vi "Test Never Any Inputs Fail.vi"(8 "error in (no error)":errorcluster, 11 "Test Case In":refnum<class "Expectation Message Test.lvclass">) -> (0 "error out":errorcluster, 3 "Test Case Out":refnum<class "Expectation Message Test.lvclass">)   [LabVIEW 2020, in "Expectation Message Test.lvclass"]
uses:
  Expectation Message Test.lvclass
  C:/Program Files (x86)/National Instruments/LabVIEW 2020/vi.lib/Astemes/LUnit/Test Case.lvclass
  Test Doubles/Test Interface Responsive Mock/Test Interface Mock.lvclass
  C:/git/astemes-lmock/source/Framework/Mock/Mock.lvclass
  source/Expectations/Never/Never Ignore Inputs.vi
  C:/git/astemes-lmock/tests/Test Doubles/Test Interface Responsive Mock/Test Interface Mock.lvclass
  C:/git/astemes-lmock/tests/Test Doubles/Test Interface/Test Interface.lvclass
  source/Framework/LMock API.lvlib
  source/Expectations/Never/Never.lvlib
  Expectation Test/Expectation Test.lvclass
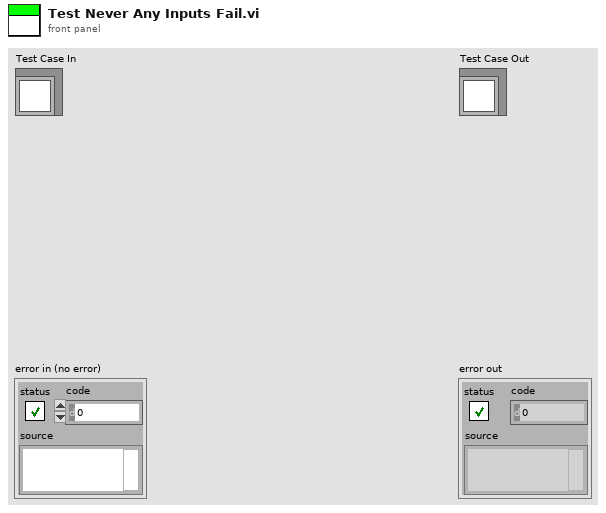
[diagram p1: front panel]
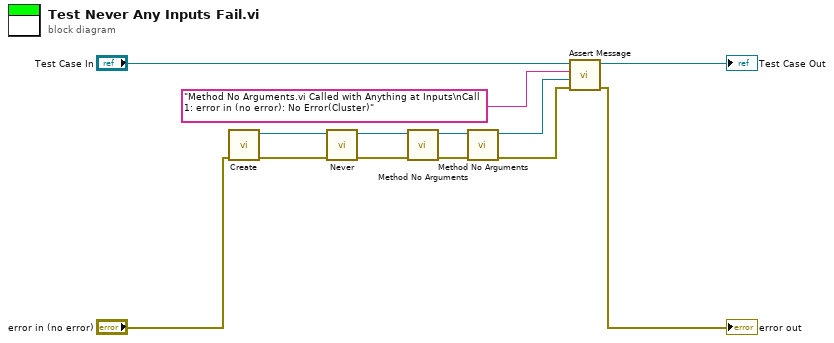
[diagram p0: block diagram]
diagram:
  n1 = call "Create.vi"("error in (no error)"="error in (no error)") -> ("error out"=w10:errorcluster, "Test Interface Mock Out"=w8:refnum<class "Test Interface Mock.lvclass">)  [unwired: 9 in]
  n2 = call-poly "Never.vi"("error in (no error)"=w10, "Mock in"=w8) -> ("error out"=w9:errorcluster, "Mock out"=w7:refnum<class "Test Interface Mock.lvclass">)  [unwired: 8 in]
  n3 = call-dynamic "Method No Arguments.vi"("error in (no error)"=w9, "Mock In"=w7) -> ("error out"=w6:errorcluster, "Mock Out"=w2:refnum<class "Test Interface Mock.lvclass">)  [unwired: 8 in]
  n4 = call-dynamic "Method No Arguments.vi"("error in (no error)"=w6, "Mock In"=w2) -> ("error out"=w3:errorcluster, "Mock Out"=w1:refnum<class "Test Interface Mock.lvclass">)  [unwired: 8 in]
  n5 = call "Assert Message.vi"("error in (no error)"=w3, "Mock"=w1, "Message"="Method No Arguments.vi Called with Anything at Inputs\nCall 1: error in (no error): No Error(Cluster)", "LUnit Test Case In"="Test Case In") -> ("error out"=→"error out":errorcluster, "LUnit Test Case Out"=→"Test Case Out":refnum<class "Expectation Message Test.lvclass">)  [unwired: 6 in]
